vi "async metadata event code.vi"(8 "error in (no error)":errorcluster, 10 "event_code_out":u32(ring)=1 items=["UHD_ASYNC_METADATA_EVENT_CODE_BURST_ACK"=1, "UHD_ASYNC_METADATA_EVENT_CODE_UNDERFLOW"=2, "UHD_ASYNC_METADATA_EVENT_CODE_SEQ_ERROR"=4, "UHD_ASYNC_METADATA_EVENT_CODE_TIME_ERROR"=8, "UHD_ASYNC_METADATA_EVENT_CODE_UNDERFLOW_IN_PACKET"=16, "UHD_ASYNC_METADATA_EVENT_CODE_SEQ_ERROR_IN_BURST"=32, "UHD_ASYNC_METADATA_EVENT_CODE_USER_PAYLOAD"=64], 11 "h":u64) -> (0 "error out":errorcluster, 1 "function return":u32(ring), 2 "event_code_out out":u32(ring)=1 items=["UHD_ASYNC_METADATA_EVENT_CODE_BURST_ACK"=1, "UHD_ASYNC_METADATA_EVENT_CODE_UNDERFLOW"=2, "UHD_ASYNC_METADATA_EVENT_CODE_SEQ_ERROR"=4, "UHD_ASYNC_METADATA_EVENT_CODE_TIME_ERROR"=8, "UHD_ASYNC_METADATA_EVENT_CODE_UNDERFLOW_IN_PACKET"=16, "UHD_ASYNC_METADATA_EVENT_CODE_SEQ_ERROR_IN_BURST"=32, "UHD_ASYNC_METADATA_EVENT_CODE_USER_PAYLOAD"=64], 3 "h out":u64)   [LabVIEW 2023, in "uhd.lvlib"]
doc: "UHD_API uhd_error uhd_async_metadata_event_code(\n uhd_async_metadata_handle h, uhd_async_metadata_event_code_t* event_code_out);"
uses:
  <userlib>/uhd/uhd.lvlib
  <userlib>/uhd/uhd.dll
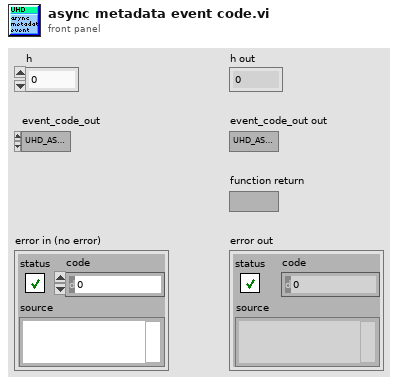
[diagram p1: front panel]
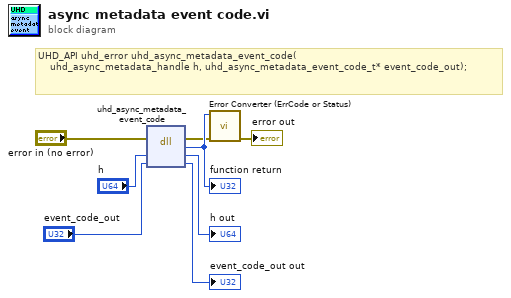
[diagram p0: block diagram]
diagram:
  # "UHD_API uhd_error uhd_async_metadata_event_code(\n    uhd_async_metadata_handle h, uhd_async_metadata_event_code_t* event_code_out);"
  n1 = dll-call lib="C:/Program Files/National Instruments/LabVIEW 2023/user.lib/uhd/uhd.*" fn="uhd_async_metadata_event_code"(error in="error in (no error)", "h"="h", "event_code_out"="event_code_out") -> (error out=w2:errorcluster, w8:u32, "h"=→"h out":u64, "event_code_out"=→"event_code_out out":u32)  [unwired: 2 in, 1 out]
  "function return" <- w8
  n2 = call <userlib>:"Error Converter (ErrCode or Status).vi"("error in (no error)"=w2, "error code"=w8) -> ("error out"=→"error out":errorcluster)  [unwired: 9 in]
